vi "Database_MLFB_Insert.vi"(3 "error in":errorcluster, 4 "Language":T2, 5 "MLFB_Info":T3, 6 "connection reference":T1) -> (0 "error out":errorcluster, 1 "Message":string, 2 "connection reference out":T1)   [LabVIEW 2015]
uses:
  CustomControl/MLFB Info.ctl
  CustomControl/Lang_Control.ctl
  <vilib>/addons/database/Connection.llb/Conn ObjectReference.ctl
  <vilib>/addons/database/NI_Database_API.lvlib
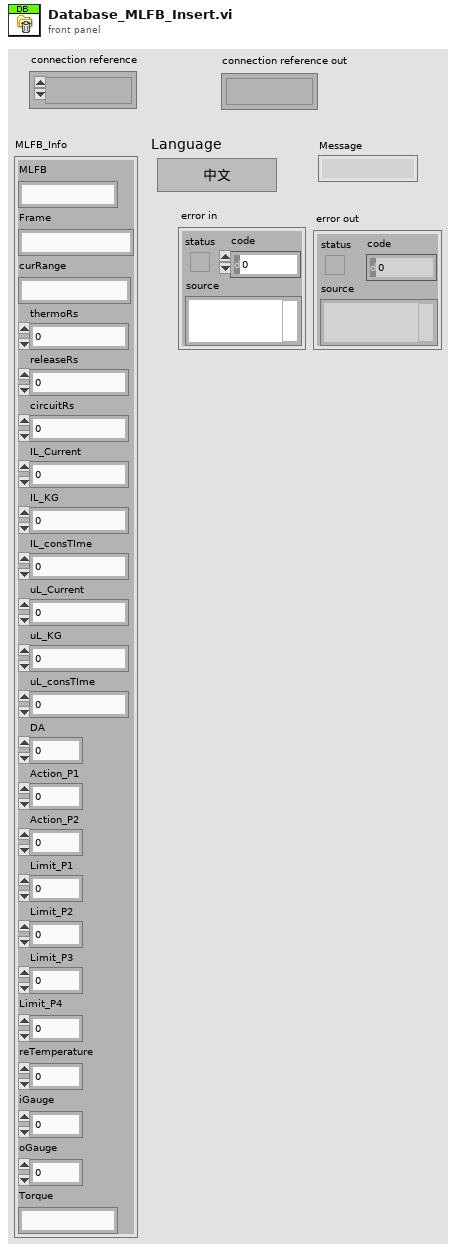
[diagram p1: front panel]
types:
  T1 = typedef "NI_Database_API.lvlib/Conn ObjectReference.ctl" = refnum<k1>
  T2 = typedef "Lang_Control.ctl" = enum16{"中文", "English"}
  T3 = typedef "MLFB Info.ctl" = cluster{"MLFB":string, "Frame":string, "curRange":string, "thermoRs":dbl, "releaseRs":dbl, "circuitRs":dbl, "IL_Current":dbl, "IL_KG":dbl, "IL_consTIme":i32, "uL_Current":dbl, "uL_KG":dbl, "uL_consTIme":i32, "DA":dbl, "Action_P1":i32, "Action_P2":i32, "Limit_P1":i32, "Limit_P2":i32, "Limit_P3":i32, "Limit_P4":i32, "reTemperature":i32, "iGauge":dbl, "oGauge":dbl, "Torque":string}
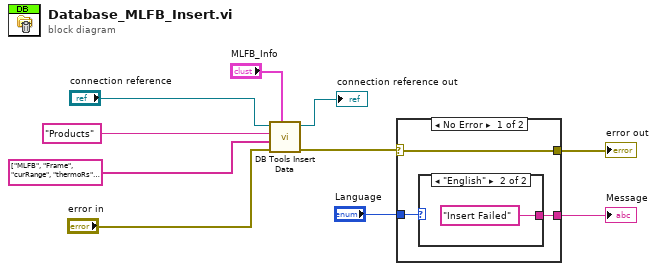
[diagram p0: block diagram]
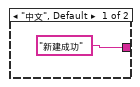
[diagram p2: hidden frame]
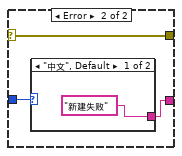
[diagram p3: hidden frame]
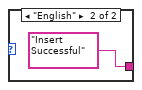
[diagram p4: hidden frame]
diagram:
  n1 = call <vilib>:"DB Tools Insert Data.vi"("data"="MLFB_Info", "error in (no error)"="error in", "columns"=string[] ["MLFB", "Frame", "curRange", "thermoRs", "releaseRs", "circuitRs", "IL_Current", "IL_KG", "IL_consTime", "uL_Current", "uL_KG", "uL_consTime", "DA", "Release_P1", "Release_P2", "Limit_P1", "Limit_P2", "Limit_P3", "Limit_P4", "reTemperature", "iGauge", "oGauge", "Torque"] ("columns 2"), "table"="Products", "connection reference"="connection reference") -> ("error out"=w2:errorcluster, "connection reference out"=→"connection reference out":T1)  [unwired: 5 in]
  n2 = case shown="No Error" w2 {
    selector: w2 -> [w13 w18]
    tunnel: [w13 w18] -> w10
    tunnel: "Language" -> [w12 w17]
    tunnel: [w11 w16] -> w6
    frame No Error {
      n3 = case shown="\"English\"" w12 {
        tunnel: ["新建成功" "Insert Failed"] -> w11
        frame "中文", Default {
        }
        frame "English" {
        }
      }
    }
    frame Error {
      n4 = case shown="\"中文\", Default" w17 {
        tunnel: ["新建失败" "Insert Successful"] -> w16
        frame "中文", Default {
        }
        frame "English" {
        }
      }
    }
  }
  "error out" <- w10
  "Message" <- w6
